vi "Update Status.vi"(8 "error in (no error)":errorcluster, 11 "Plugin in":refnum<class "Plugin.lvclass">) -> (0 "error out":errorcluster, 3 "Plugin out":refnum<class "Plugin.lvclass">)   [LabVIEW 2017, in "DSF Core.lvlib" / "Plugin.lvclass"]
uses:
  Plugin.lvclass
  Plugin.lvclass/Plugin.ctl
  Status/Status Data.ctl
  Status/Status.lvclass
  Timing/Timing.lvclass
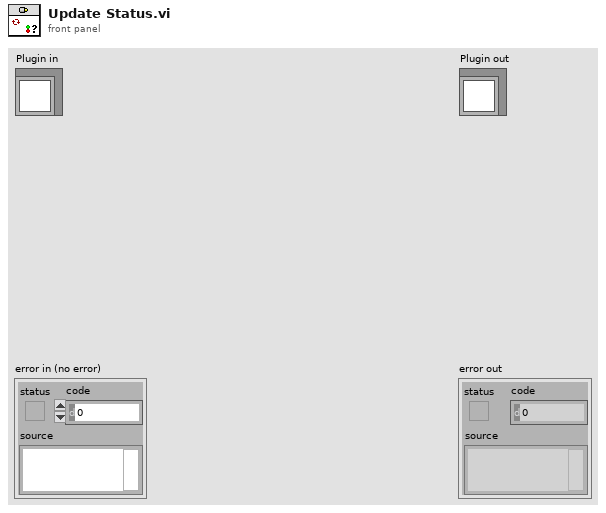
[diagram p1: front panel]
types:
  T1 = typedef "DSF Core.lvlib/Status.lvclass/Status Data.ctl" = cluster{"late count":u64, "iteration":u64, "duration":u32}
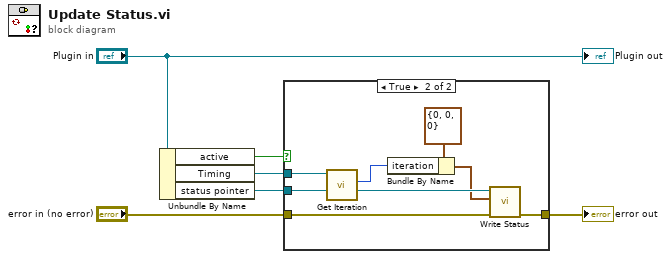
[diagram p0: block diagram]
diagram:
  n1 = Unbundle By Name("Plugin in") -> ("active"=w1:bool, "Timing"=w6:refnum<class "Timing.lvclass">, "status pointer"=w5:refnum<class "Status.lvclass">)
  n2 = case shown="True" w1 {
    tunnel: w6 -> [_ w13]
    tunnel: w5 -> [_ w12]
    tunnel: "error in (no error)" -> [w7 w10]
    tunnel: [w7 w9] -> w3
    frame False {
    }
    frame True {
      n3 = call "Get Iteration.vi"("Timing in"=w13) -> ("Iteration"=w11:u64)  [unwired: 9 in, 1 out]
      n4 = Bundle By Name(cluster=T1 {"late count"=0, "iteration"=0, "duration"=0} ("status"), "iteration"=w11) -> (w8:T1)
      n5 = call "Write Status.vi"("error in (no error)"=w10, "status"=w8, "status pointer in"=w12) -> ("error out"=w9:errorcluster)  [unwired: 7 in, 1 out]
    }
  }
  "error out" <- w3
  "Plugin out" <- "Plugin in"
